vi "Change_Leak_Comp_Mode.vi"(8 "error in (no error)":errorcluster) -> (0 "error out":errorcluster, 3 "LeakCompMode":dbl)   [LabVIEW 2020]
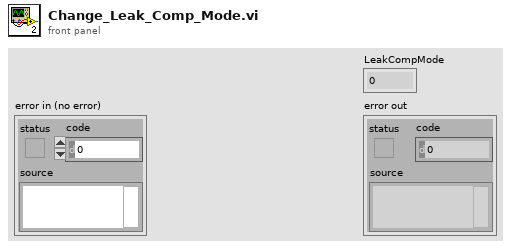
[diagram p1: front panel]
types:
  T1 = enum16{"Left Button", "Center Button", "Right Button", "Window Close"}
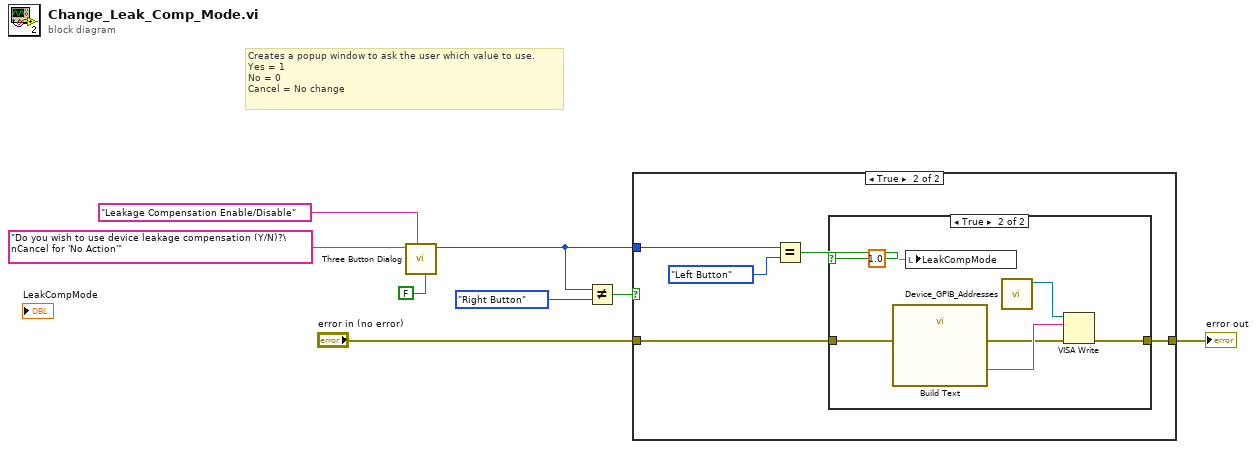
[diagram p0: block diagram]
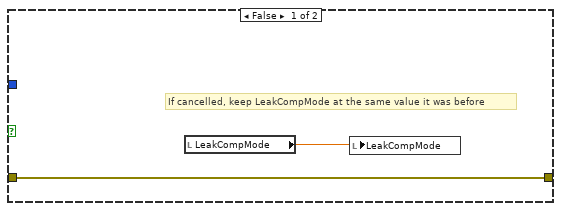
[diagram p2: hidden frame]
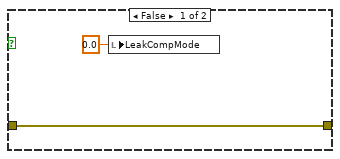
[diagram p3: hidden frame]
diagram:
  # "Creates a popup window to ask the user which value to use.\nYes = 1\nNo = 0\nCancel = No change"
  n1 = call <vilib>:"Three Button Dialog.vi"("Allow user to close window? (TRUE)"=FALSE, "Window Title (\"\")"="Leakage Compensation Enable/Disable" ("Window Title (\"\")"), "message"="Do you wish to use device leakage compensation (Y/N)?\nCancel for 'No Action'") -> ("Which Button?"=w2:T1)  [unwired: 8 in]
  n2 = Not Equal?(x=w2, y=T1."Right Button") -> (x != y?=w1:bool)
  n3 = case shown="True" w1 {
    tunnel: "error in (no error)" -> [w10 w14]
    tunnel: w2 -> [_ w13]
    tunnel: [w10 w11] -> w4
    frame False {
      # "If cancelled, keep LeakCompMode at the same value it was before"
      n4 = local read "LeakCompMode"() -> (w9:dbl)
      n5 = local write "LeakCompMode"(w9) -> ()
    }
    frame True {
      n6 = Equal?(x=w13, y=T1."Left Button") -> (x = y?=w15:bool)
      n7 = case shown="True" w15 {
        tunnel: w14 -> [w16 w22]
        tunnel: [w16 w18] -> w11
        frame False {
          n8 = local write "LeakCompMode"(0.0 ("LeakCompMode")) -> ()
        }
        frame True {
          n9 = call "Build Text"("error in (no error)"=w22) -> ("Result"=w20:string, "error out"=w19:errorcluster)  [unwired: 13 in]
          n10 = local write "LeakCompMode"(1.0) -> ()
          n11 = call "Device_GPIB_Addresses.vi"() -> ("Keithley 2400 Address"=w21:refnum<visa-resource-name>)  [unwired: 9 in, 2 out]
          n12 = VISA Write(VISA resource name=w21, write buffer=w20, error in (no error)=w19) -> (error out=w18:errorcluster)  [unwired: 2 out]
        }
      }
    }
  }
  "error out" <- w4
